vi "subCalculateSpecificationBuildOrder.vi"(6 "UpdateList":refnum<user-event>, 8 "error in (no error)":errorcluster, 11 "Item info":T2) -> (0 "error out":errorcluster, 3 "Dependency order":T1[](array[typedef]))   [LabVIEW 2020, in "SolutionBuilder.lvlib"]
uses:
  SolutionBuilder.lvlib
  ItemInfo.ctl
  ProjectInfo.ctl
  FileInfo.ctl
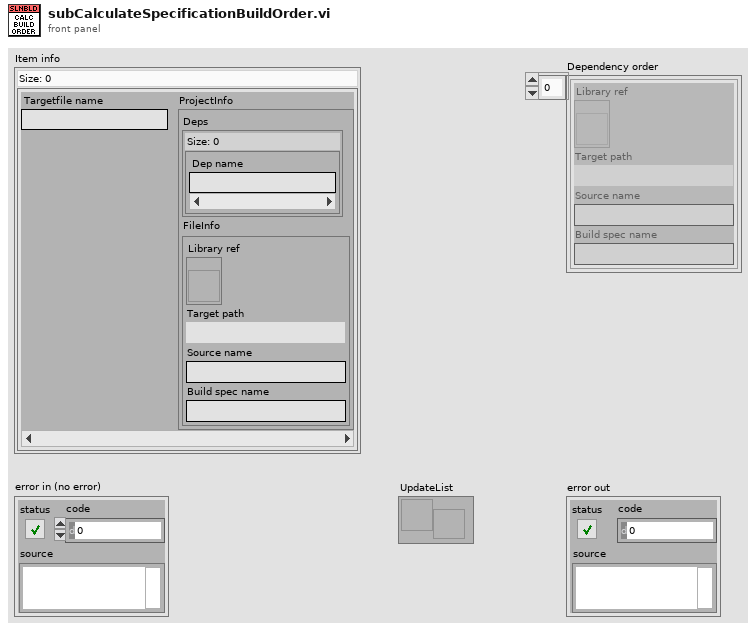
[diagram p1: front panel]
types:
  T1 = typedef "SolutionBuilder.lvlib/FileInfo.ctl" = cluster{"Library ref":refnum<vi>, "Target path":path, "Source name":string, "Build spec name":string}
  T2 = typedef "SolutionBuilder.lvlib/ItemInfo.ctl" = map{string, T3}
  T3 = typedef "SolutionBuilder.lvlib/ProjectInfo.ctl" = cluster{"Deps":set{string}, "FileInfo":T1}
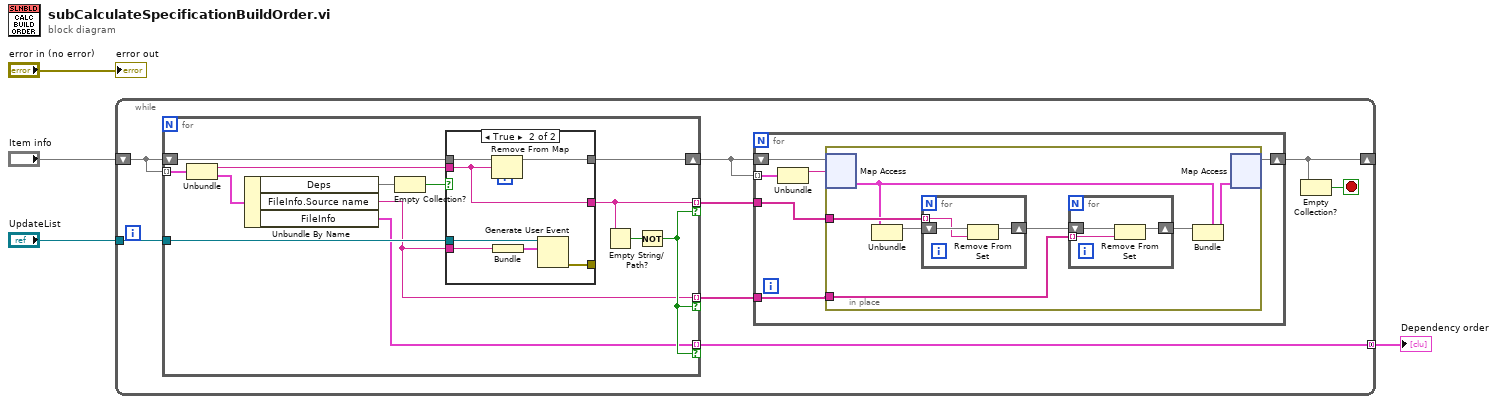
[diagram p0: block diagram]
diagram:
  n1 = while {
    shift-right: [w7] -> _
    shift-left: "Item info" -> [w12]
    tunnel: [w10] -> w1 mode=concatenating
    tunnel: "UpdateList" -> [w6]
    stop <- w11 stop-if-true
    n2 = for {
      tunnel: w12 -> [w25] mode=indexing
      shift-right: [w21] -> w9
      shift-left: w12 -> [w22]
      tunnel: [w14] -> w10 mode=indexing if=w17
      tunnel: [w18] -> w8 mode=indexing if=w17
      tunnel: w6 -> [w19]
      tunnel: [w13] -> w5 mode=indexing if=w17
      n3 = Unbundle(w25) -> ("Targetfile name"=w24:string, "ProjectInfo"=w16:T3)
      n4 = Unbundle By Name(w16) -> ("Deps"=w15:set{string}, "FileInfo.Source name"=w13:string, "FileInfo"=w14:T1)
      n5 = Empty Collection?(1:w15) -> (0:w23:bool)
      n6 = case shown="True" w23 {
        tunnel: w24 -> [_ w31]
        tunnel: w22 -> [w26 w33]
        tunnel: [w26 w32] -> w21
        tunnel: [_ w31] -> w18
        tunnel: w19 -> [_ w28]
        tunnel: [_ w29] -> _
        tunnel: w13 -> [_ w27]
        frame False {
        }
        frame True {
          n7 = Remove From Map(10:w31, 11:w33) -> (3:w32:T2)  [unwired: 2 out]
          n8 = Bundle("Source name"=w27) -> (w30:cluster{"Source name":string})  [unwired: 1 in]
          n9 = Generate User Event(user event=w28, event data cluster=w30) -> (error out=w29:errorcluster)  [unwired: 2 in, 1 out]
        }
      }
      n10 = Empty String/Path?(string/path=w18) -> (empty?=w20:bool)
      n11 = Not(x=w20) -> (.not. x?=w17:bool)
    }
    n12 = for {
      shift-right: [w35] -> w7
      shift-left: w9 -> [w38]
      tunnel: w9 -> [w39] mode=indexing
      tunnel: w8 -> [w36]
      tunnel: w5 -> [w34]
      n13 = Unbundle(w39) -> ("Targetfile name"=w37:string)  [unwired: 1 out]
      n14 = in-place {
        in-place-border: w36 -> [w45]
        in-place-border: w34 -> [w40]
        n15 = in-place-map #1(w38, w37) -> (w44:T3)  [unwired: 1 in, 1 out]
        n16 = Unbundle(w44) -> ("Deps"=w46:set{string})  [unwired: 1 out]
        n17 = for {
          tunnel: w45 -> [w51] mode=indexing
          shift-right: [w50] -> w42
          shift-left: w46 -> [w52]
          n18 = Remove From Set(10:w51, 11:w52) -> (3:w50:set{string})  [unwired: 1 out]
        }
        n19 = for {
          tunnel: w40 -> [w48] mode=indexing
          shift-right: [w47] -> w41
          shift-left: w42 -> [w49]
          n20 = Remove From Set(10:w48, 11:w49) -> (3:w47:set{string})  [unwired: 1 out]
        }
        n21 = Bundle(cluster=w44, "Deps"=w41) -> (w43:T3)  [unwired: 1 in]
        n22 = in-place-map #1(w43) -> (w35:T2)  [unwired: 1 in, 2 out]
      }
    }
    n23 = Empty Collection?(1:w7) -> (0:w11:bool)
  }
  "Dependency order" <- w1
  "error out" <- "error in (no error)"
